vi "Keep Alive Count.vi"(11 "RequestTraceLog in":refnum<class "RequestTraceLog.lvclass">) -> (2 "Keep Alive Count":i32, 3 "RequestTraceLog out":refnum<class "RequestTraceLog.lvclass">)   [LabVIEW 2020, in "HTTP Server.lvlib" / "RequestTraceLog.lvclass"]
uses:
  RequestTraceLog.lvclass
  RequestTraceLog.lvclass/RequestTraceLog.ctl
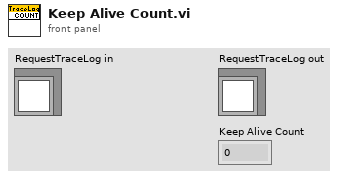
[diagram p1: front panel]
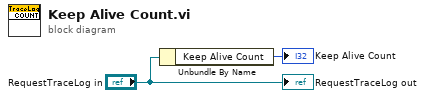
[diagram p0: block diagram]
diagram:
  n1 = Unbundle By Name("RequestTraceLog in") -> ("Keep Alive Count"=→"Keep Alive Count":i32)
  "RequestTraceLog out" <- "RequestTraceLog in"
